vi "Counter - Continuous Output.vi"() -> ()   [LabVIEW 2021]
doc: "This example demonstrates how to continuously generate digital pulses using a counter output."
uses:
  <vilib>/Utility/error.llb/DialogType.ctl
  <vilib>/DAQmx/create/channels.llb/DAQmx Create Channel (CO-Pulse Generation-Frequency).vi
  <vilib>/DAQmx/configure/timing.llb/DAQmx Timing (Implicit).vi
  <vilib>/DAQmx/configure/trigger.llb/DAQmx Start Trigger (Digital Edge).vi
  <resource>/objmgr/daqmx.rc
panel:
  out "Actual Duty Cycle":dbl
  out "Actual Frequency":dbl
  in  "Duty Cycle":dbl=0.5 format="%.6f"
  in  "Frequency":dbl=1.0 format="%.6f"
  in  "Output Terminal":tag="/Dev1/PFI12"
  in  "Trigger Type":T1(tab)
  in  "Edge":i32(ring)=10280 items=["Rising"=10280, "Falling"=10171]
  in  "Digital Trigger Source":tag
  in  "Pause When":i32(ring)=10192 items=["High"=10192, "Low"=10214]
  in  "Pause Trigger Source":tag
  in  "Stop":bool
  in  "Counter":tag="Dev1/ctr0"
  # "Channel Settings"
  # "Trigger Settings"
  # "To configure and use a trigger you must have the necessary tab selected above."
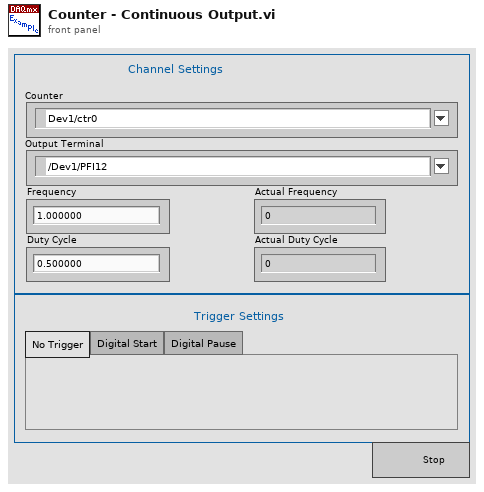
[diagram p1: front panel]
types:
  T1 = enum32{"No Trigger", "Digital Start", "Digital Pause"}
  T2 = typedef "DialogType.ctl" = u16
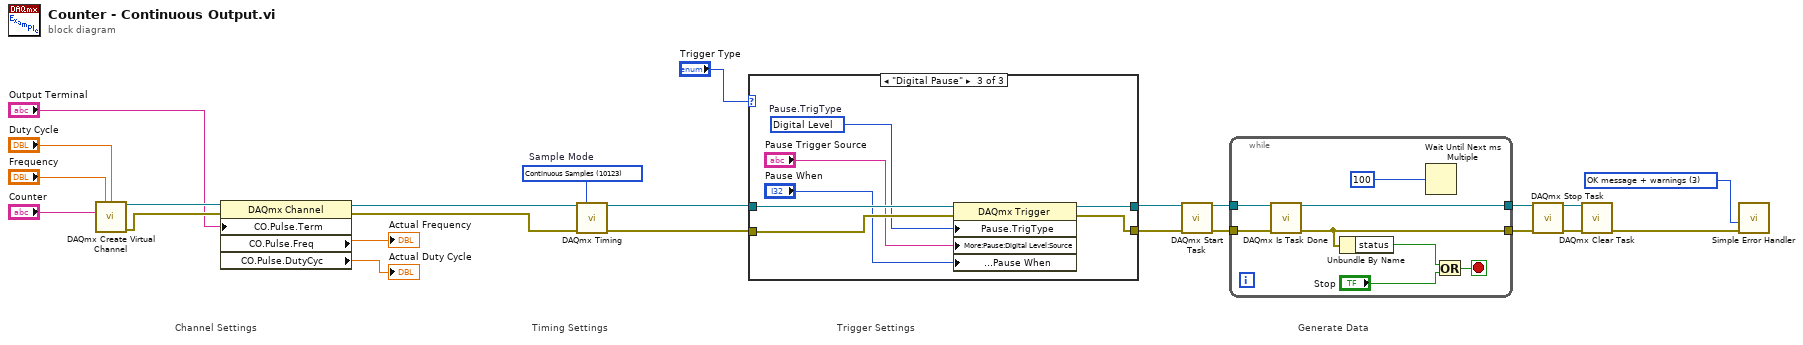
[diagram p0: block diagram]
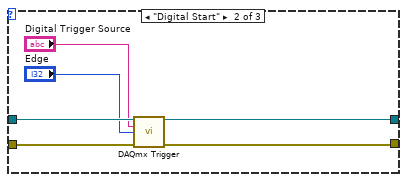
[diagram p3: hidden frame]
diagram:
  w1 = T2 3 items=["no dialog", "OK message", "continue or stop message", "OK message + warnings", "continue/stop + warnings"] ("type of dialog (OK msg:1)")
  w24 = 10123 items=["Finite Samples"=10178, "Continuous Samples"=10123, "Hardware Timed Single Point"=12522]  # Sample Mode
  # "Generate Data"
  # "Trigger Settings"
  # "Timing Settings"
  # "Channel Settings"
  n1 = call-poly <vilib>:"DAQmx Create Virtual Channel.vi"("frequency"="Frequency", "duty cycle"="Duty Cycle", "counter"="Counter") -> ("task out"=w14:refnum<k21>, "error out"=w13:errorcluster)  [unwired: 11 in]
  n2 = property class="DAQmx Channel"(reference=w14, error in=w13, "CO.Pulse.Term"="Output Terminal") -> (reference out=w10:refnum<k21>, error out=w11:errorcluster, "CO.Pulse.Freq"=→"Actual Frequency":dbl, "CO.Pulse.DutyCyc"=→"Actual Duty Cycle":dbl)
  n3 = call-poly <vilib>:"DAQmx Timing.vi"("task/channels in"=w10, "sample mode"=w24, "error in"=w11) -> ("task out"=w18:refnum<k21>, "error out"=w17:errorcluster)  [unwired: 11 in]
  n4 = case shown="\"Digital Pause\"" "Trigger Type" {
    tunnel: w18 -> [w26 w32 w39]
    tunnel: w17 -> [w25 w31 w36]
    tunnel: [w26 w30 w38] -> w15
    tunnel: [w25 w29 w37] -> w16
    frame "No Trigger", Default {
    }
    frame "Digital Start" {
      n5 = call-poly <vilib>:"DAQmx Trigger.vi"("task/channels in"=w32, "source"="Digital Trigger Source", "edge"="Edge", "error in"=w31) -> ("task out"=w30:refnum<k21>, "error out"=w29:errorcluster)  [unwired: 10 in]
    }
    frame "Digital Pause" {
      w35 = 10152 items=["Analog Level"=10101, "Analog Window"=10103, "Digital Level"=10152, "Digital Pattern"=10398, "None"=10230]  # Pause.TrigType
      n6 = property class="DAQmx Trigger"(reference=w39, error in=w36, "Pause.TrigType"=w35, "More:Pause:Digital Level:Source"="Pause Trigger Source", "More:Pause:Digital Level:Pause When"="Pause When") -> (reference out=w38:refnum<k21>, error out=w37:errorcluster)
    }
  }
  n7 = call <vilib>:"DAQmx Start Task.vi"("task/channels in"=w15, "error in"=w16) -> ("task out"=w23:refnum<k21>, "error out"=w22:errorcluster)  [unwired: 12 in]
  n8 = while {
    tunnel: w23 -> [w47]
    tunnel: w22 -> [w46]
    tunnel: [w43] -> w2
    tunnel: [w44] -> w3
    stop <- w45 stop-if-true
    n9 = call <vilib>:"DAQmx Is Task Done.vi"("task/channels in"=w47, "error in"=w46) -> ("task out"=w44:refnum<k21>, "error out"=w43:errorcluster)  [unwired: 11 in, 1 out]
    n10 = Unbundle By Name(w43) -> ("status"=w42:bool)
    n11 = Wait Until Next ms Multiple(millisecond multiple=u32 100) -> ()  [unwired: 1 out]
    n12 = Or(x=w42, y="Stop") -> (x .or. y?=w45:bool)
  }
  n13 = call <vilib>:"DAQmx Stop Task.vi"("task/channels in"=w3, "error in"=w2) -> ("task out"=w5:refnum<k21>, "error out"=w4:errorcluster)  [unwired: 12 in]
  n14 = call <vilib>:"DAQmx Clear Task.vi"("task in"=w5, "error in"=w4) -> ("error out"=w21:errorcluster)  [unwired: 13 in]
  n15 = call <vilib>:"Simple Error Handler.vi"("type of dialog (OK msg:1)"=w1, "error in (no error)"=w21) -> ()  [unwired: 3 in, 5 out]
